vi "Cavities_State_v00.vi"(4 "BS Hold Pulse":bool, 6 "\"I too high?\"":T11, 11 "Control Cavity Cluster":T8={"Control A"={"Lock"=FALSE, "Hold"=FALSE, "P Gain"=0, "P BS"=-5, "I Gain"=0, "I BS"=-10, "I2 G"=0, "I2 BS"=-26, "Scan Amp"=0, "Scan Off"=0, "Scan FS"=0, "SFS BS"=0, "I Max value"=10000, "I2 Max value"=10000, "Scope.Offset"=0, "Trigger Direction"=enum."either", "Scan-PII thresh"=0}, "Control B"={"Lock"=FALSE, "Hold"=FALSE, "P Gain"=0, "P BS"=-5, "I Gain"=0, "I BS"=-10, "I2 G"=0, "I2 BS"=-26, "Scan Amp"=0, "Scan Off"=0, "Scan FS"=0, "SFS BS"=0, "I Max value"=10000, "I2 Max value"=10000, "Scope.Offset"=0, "Trigger Direction"=enum."either", "Scan-PII thresh"=0}, "Control MCC"={"Lock"=FALSE, "Hold"=FALSE, "P Gain"=0, "P BS"=-5, "I Gain"=0, "I BS"=-10, "I2 G"=0, "I2 BS"=-26, "Scan Amp"=0, "Scan Off"=0, "Scan FS"=0, "SFS BS"=0, "I Max value"=10000, "I2 Max value"=10000, "Scope.Offset"=0, "Trigger Direction"=enum."either", "Scan-PII thresh"=0}, "Control Doubler"={"Lock"=FALSE, "Hold"=FALSE, "P Gain"=0, "P BS"=-5, "I Gain"=0, "I BS"=-10, "I2 G"=0, "I2 BS"=-26, "Scan Amp"=0, "Scan Off"=0, "Scan FS"=0, "SFS BS"=0, "I Max value"=10000, "I2 Max value"=10000, "Scope.Offset"=0, "Trigger Direction"=enum."either", "Scan-PII thresh"=0}, "Lock Point?"={"OPO A"=FALSE, "OPO B"=FALSE, "MCC"=FALSE, "Doubler"=FALSE}, "Re-scan?"={"OPO A"=FALSE, "OPO B"=FALSE, "MCC"=FALSE, "Doubler"=FALSE}, "Cavity Errors"={"OPO A"=0, "OPO B"=0, "MCC"=0, "Doubler"=0}, "Max"={"Max OPO A"=0, "Max OPO B"=0, "Max MCC"=0, "Max Doubler"=0}, "Min"={"Min OPO A"=0, "Min OPO B"=0, "Min MCC"=0, "Min Doubler"=0}, "Lock Threshold"={"Thresh OPO A "=0, "Thresh OPO B"=0, "Thresh MCC"=0, "Thresh Doubler"=0}, "Re-Scan Threshold"={"Thresh OPO A "=0, "Thresh OPO B"=0, "Thresh MCC"=0, "Thresh Doubler"=0}, "State (-1)"={"OPO A"=enum."Safe", "OPO B"=enum."Safe", "MCC"=enum."Safe", "Doubler"=enum."Safe"}, "Lock pressed? (-1)"={"OPO A"=FALSE, "OPO B"=FALSE, "MCC"=FALSE, "Doubler"=FALSE}, "Safety First"={"lim reset"=FALSE, "no limit"=FALSE, "pos slew rate * dt"=0, "neg slew rate * dt"=0, "Hold All"=FALSE, "Count(Ticks)"=0}}) -> (3 "PII Scan State Errors":T5={"Control A"={"Lock"=FALSE, "Hold"=FALSE, "P Gain"=3, "P BS"=0, "I Gain"=0, "I BS"=-10, "I2 G"=0, "I2 BS"=-26, "Scan Amp"=0, "Scan Off"=0, "Scan FS"=0, "SFS BS"=0, "I Max value"=10000, "I2 Max value"=10000, "Scope.Offset"=0, "Trigger Direction"=enum."either", "Scan-PII thresh"=0}, "Control B"={"Lock"=FALSE, "Hold"=FALSE, "P Gain"=0, "P BS"=-5, "I Gain"=0, "I BS"=-10, "I2 G"=0, "I2 BS"=-26, "Scan Amp"=0, "Scan Off"=0, "Scan FS"=0, "SFS BS"=0, "I Max value"=10000, "I2 Max value"=10000, "Scope.Offset"=0, "Trigger Direction"=enum."either", "Scan-PII thresh"=0}, "Control MCC"={"Lock"=FALSE, "Hold"=FALSE, "P Gain"=0, "P BS"=-5, "I Gain"=0, "I BS"=-10, "I2 G"=0, "I2 BS"=-26, "Scan Amp"=0, "Scan Off"=0, "Scan FS"=0, "SFS BS"=0, "I Max value"=10000, "I2 Max value"=10000, "Scope.Offset"=0, "Trigger Direction"=enum."either", "Scan-PII thresh"=0}, "Control Doubler"={"Lock"=FALSE, "Hold"=FALSE, "P Gain"=0, "P BS"=-5, "I Gain"=0, "I BS"=-10, "I2 G"=0, "I2 BS"=-26, "Scan Amp"=0, "Scan Off"=0, "Scan FS"=0, "SFS BS"=0, "I Max value"=10000, "I2 Max value"=10000, "Scope.Offset"=0, "Trigger Direction"=enum."either", "Scan-PII thresh"=0}, "Cavity Errors"={"OPO A"=0, "OPO B"=0, "MCC"=0, "Doubler"=0}, "State"={"OPO A"=enum."Safe", "OPO B"=enum."Safe", "MCC"=enum."Safe", "Doubler"=enum."Safe"}}, 5 "MaxMin":T1)   [LabVIEW 2010]
doc: "The state of the output is decided here. There are four possible states: 1) Safe - zeros; 2) Hold - constant output of last value; 3) Scan - saw tooth at low frequency 4) Lock - PII output."
uses:
  Strict Type Defs/PII Scan State.ctl
  Strict Type Defs/PII individual.ctl
  Strict Type Defs/Cavity Errors.ctl
  Strict Type Defs/Control Cavity Cluster.ctl
  Strict Type Defs/Lock Point.ctl
  Strict Type Defs/Re-Scan.ctl
  Strict Type Defs/Max.ctl
  Strict Type Defs/Min.ctl
  Strict Type Defs/Safety First.ctl
  Strict Type Defs/MaxMin.ctl
panel:
  in  "MaxMin typedef":T1
  in  "Lock?":T11
  in  "PII Scan State":T5={"Control A"={"Lock"=FALSE, "Hold"=FALSE, "P Gain"=3, "P BS"=0, "I Gain"=0, "I BS"=-10, "I2 G"=0, "I2 BS"=-26, "Scan Amp"=0, "Scan Off"=0, "Scan FS"=0, "SFS BS"=0, "I Max value"=10000, "I2 Max value"=10000, "Scope.Offset"=0, "Trigger Direction"=enum."either", "Scan-PII thresh"=0}, "Control B"={"Lock"=FALSE, "Hold"=FALSE, "P Gain"=0, "P BS"=-5, "I Gain"=0, "I BS"=-10, "I2 G"=0, "I2 BS"=-26, "Scan Amp"=0, "Scan Off"=0, "Scan FS"=0, "SFS BS"=0, "I Max value"=10000, "I2 Max value"=10000, "Scope.Offset"=0, "Trigger Direction"=enum."either", "Scan-PII thresh"=0}, "Control MCC"={"Lock"=FALSE, "Hold"=FALSE, "P Gain"=0, "P BS"=-5, "I Gain"=0, "I BS"=-10, "I2 G"=0, "I2 BS"=-26, "Scan Amp"=0, "Scan Off"=0, "Scan FS"=0, "SFS BS"=0, "I Max value"=10000, "I2 Max value"=10000, "Scope.Offset"=0, "Trigger Direction"=enum."either", "Scan-PII thresh"=0}, "Control Doubler"={"Lock"=FALSE, "Hold"=FALSE, "P Gain"=0, "P BS"=-5, "I Gain"=0, "I BS"=-10, "I2 G"=0, "I2 BS"=-26, "Scan Amp"=0, "Scan Off"=0, "Scan FS"=0, "SFS BS"=0, "I Max value"=10000, "I2 Max value"=10000, "Scope.Offset"=0, "Trigger Direction"=enum."either", "Scan-PII thresh"=0}, "Cavity Errors"={"OPO A"=0, "OPO B"=0, "MCC"=0, "Doubler"=0}, "State"={"OPO A"=enum."Safe", "OPO B"=enum."Safe", "MCC"=enum."Safe", "Doubler"=enum."Safe"}}
  in  "State":T12
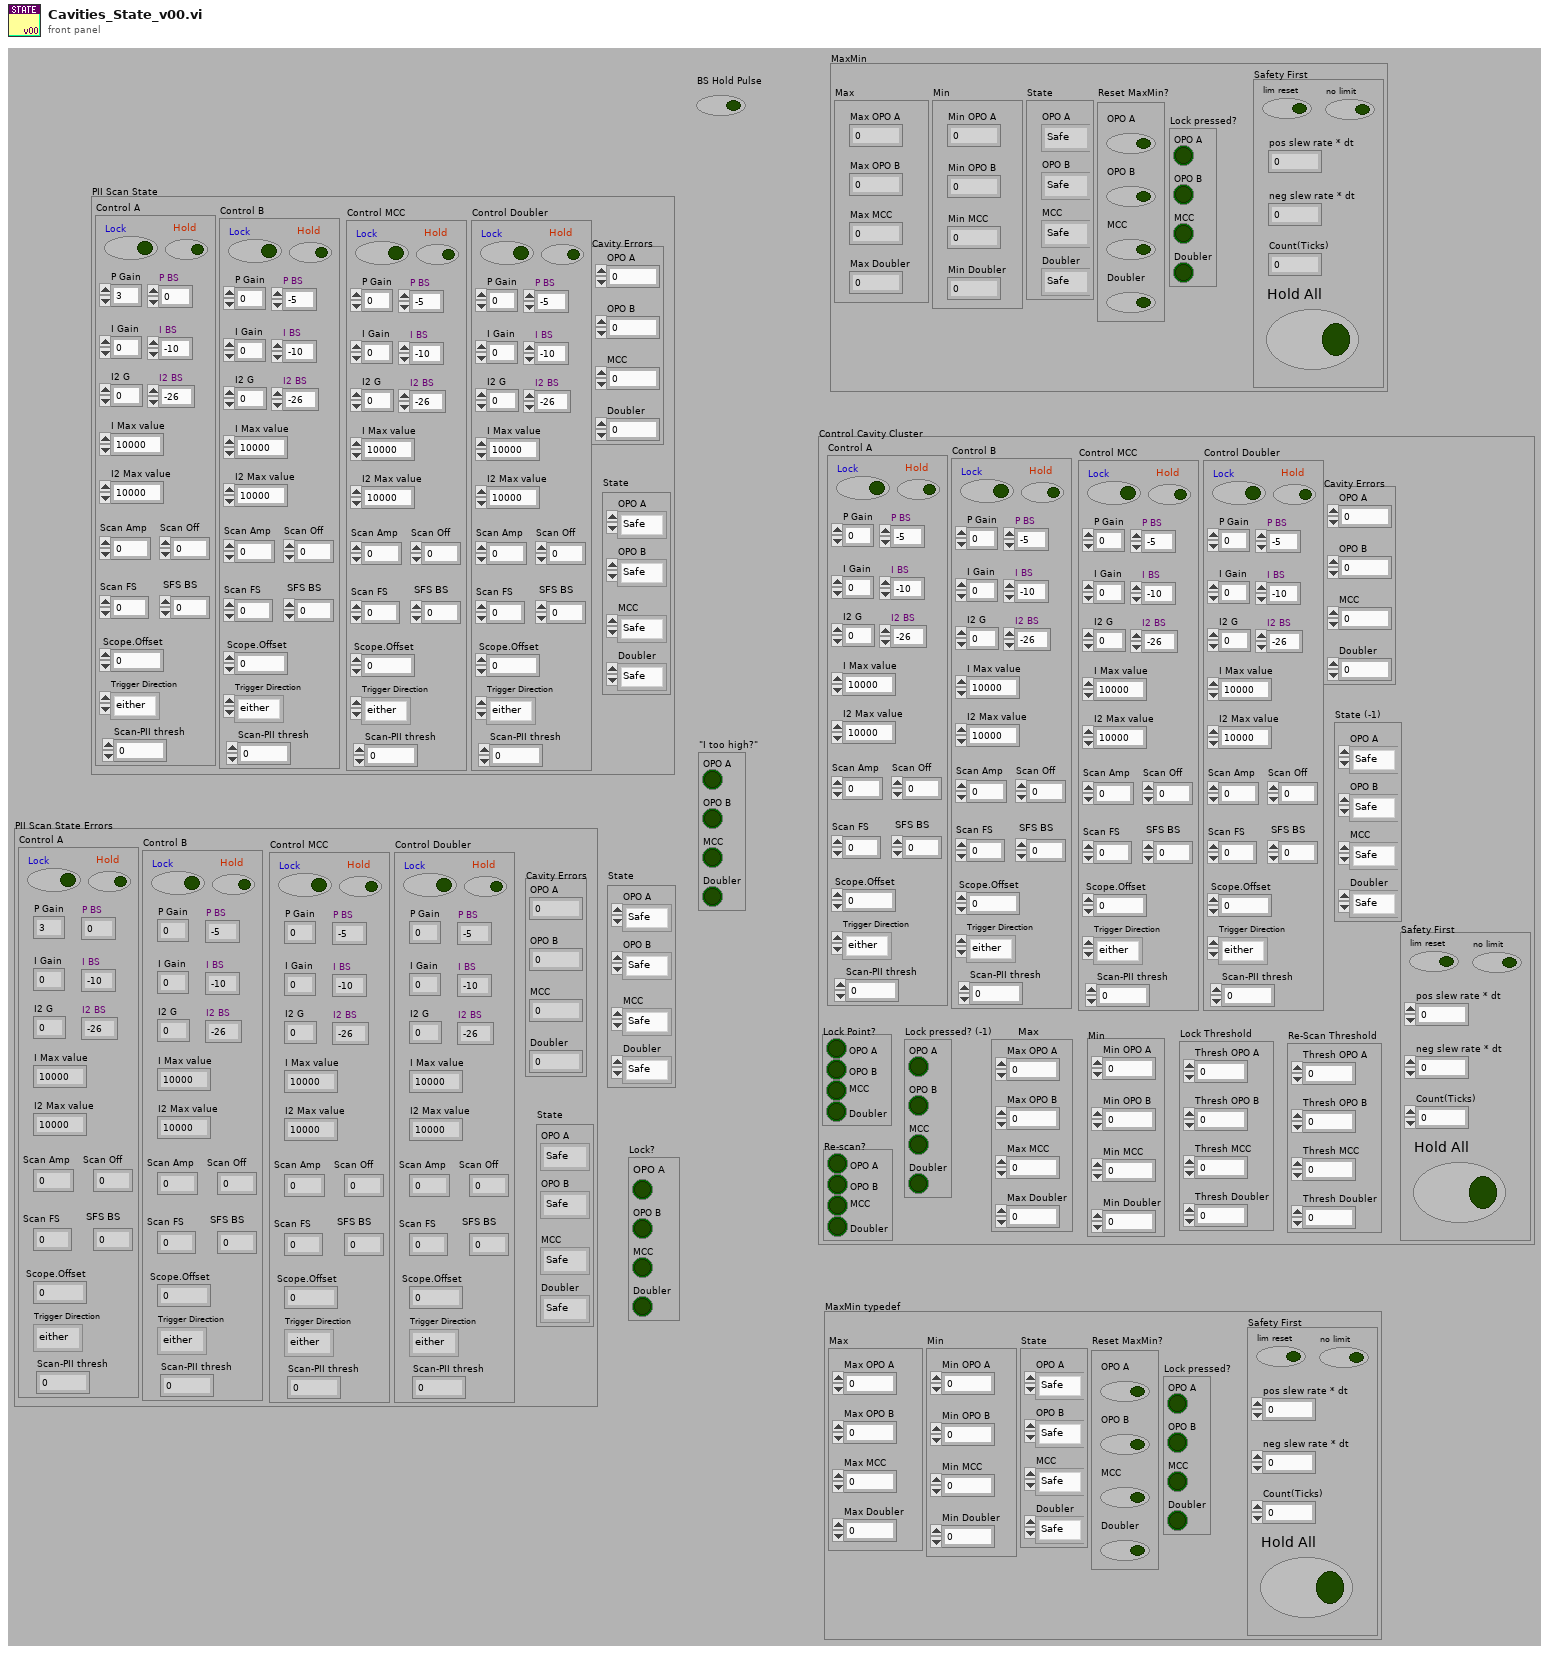
[diagram p1: front panel]
types:
  T1 = typedef "MaxMin.ctl" = cluster{"State":cluster{"OPO A":enum16{"Safe", "Hold", "Scan", "Lock"}, "OPO B":enum16{"Safe", "Hold", "Scan", "Lock"}, "MCC":enum16{"Safe", "Hold", "Scan", "Lock"}, "Doubler":enum16{"Safe", "Hold", "Scan", "Lock"}}, "Reset MaxMin?":cluster{"OPO A":bool, "OPO B":bool, "MCC":bool, "Doubler":bool}, "Max":T2, "Min":T3, "Lock pressed?":cluster{"OPO A":bool, "OPO B":bool, "MCC":bool, "Doubler":bool}, "Safety First":T4}
  T2 = typedef "Max.ctl" = cluster{"Max OPO A":i16, "Max OPO B":i16, "Max MCC":i16, "Max Doubler":i16}
  T3 = typedef "Min.ctl" = cluster{"Min OPO A":i16, "Min OPO B":i16, "Min MCC":i16, "Min Doubler":i16}
  T4 = typedef "Safety First.ctl" = cluster{"lim reset":bool, "no limit":bool, "pos slew rate * dt":i16, "neg slew rate * dt":i16, "Hold All":bool, "Count(Ticks)":u32}
  T5 = typedef "PII Scan State.ctl" = cluster{"Control A":T6, "Control B":T6, "Control MCC":T6, "Control Doubler":T6, "Cavity Errors":T7, "State":cluster{"OPO A":enum16{"Safe", "Hold", "Scan", "Lock"}, "OPO B":enum16{"Safe", "Hold", "Scan", "Lock"}, "MCC":enum16{"Safe", "Hold", "Scan", "Lock"}, "Doubler":enum16{"Safe", "Hold", "Scan", "Lock"}}}
  T6 = typedef "PII individual.ctl" = cluster{"Lock":bool, "Hold":bool, "P Gain":i32, "P BS":i16, "I Gain":i32, "I BS":i16, "I2 G":i32, "I2 BS":i16, "Scan Amp":i16, "Scan Off":i16, "Scan FS":u16, "SFS BS":i16, "I Max value":i32, "I2 Max value":i32, "Scope.Offset":i16, "Trigger Direction":enum8{"either", "minus-plus", "plus-minus"}, "Scan-PII thresh":i16}
  T7 = typedef "Cavity Errors.ctl" = cluster{"OPO A":i16, "OPO B":i16, "MCC":i16, "Doubler":i16}
  T8 = typedef "Control Cavity Cluster.ctl" = cluster{"Control A":T6, "Control B":T6, "Control MCC":T6, "Control Doubler":T6, "Lock Point?":T9, "Re-scan?":T10, "Cavity Errors":T7, "Max":T2, "Min":T3, "Lock Threshold":cluster{"Thresh OPO A ":i16, "Thresh OPO B":i16, "Thresh MCC":i16, "Thresh Doubler":i16}, "Re-Scan Threshold":cluster{"Thresh OPO A ":i16, "Thresh OPO B":i16, "Thresh MCC":i16, "Thresh Doubler":i16}, "State (-1)":cluster{"OPO A":enum16{"Safe", "Hold", "Scan", "Lock"}, "OPO B":enum16{"Safe", "Hold", "Scan", "Lock"}, "MCC":enum16{"Safe", "Hold", "Scan", "Lock"}, "Doubler":enum16{"Safe", "Hold", "Scan", "Lock"}}, "Lock pressed? (-1)":cluster{"OPO A":bool, "OPO B":bool, "MCC":bool, "Doubler":bool}, "Safety First":T4}
  T9 = typedef "Lock Point.ctl" = cluster{"OPO A":bool, "OPO B":bool, "MCC":bool, "Doubler":bool}
  T10 = typedef "Re-Scan.ctl" = cluster{"OPO A":bool, "OPO B":bool, "MCC":bool, "Doubler":bool}
  T11 = cluster{"OPO A":bool, "OPO B":bool, "MCC":bool, "Doubler":bool}
  T12 = cluster{"OPO A":enum16{"Safe", "Hold", "Scan", "Lock"}, "OPO B":enum16{"Safe", "Hold", "Scan", "Lock"}, "MCC":enum16{"Safe", "Hold", "Scan", "Lock"}, "Doubler":enum16{"Safe", "Hold", "Scan", "Lock"}}
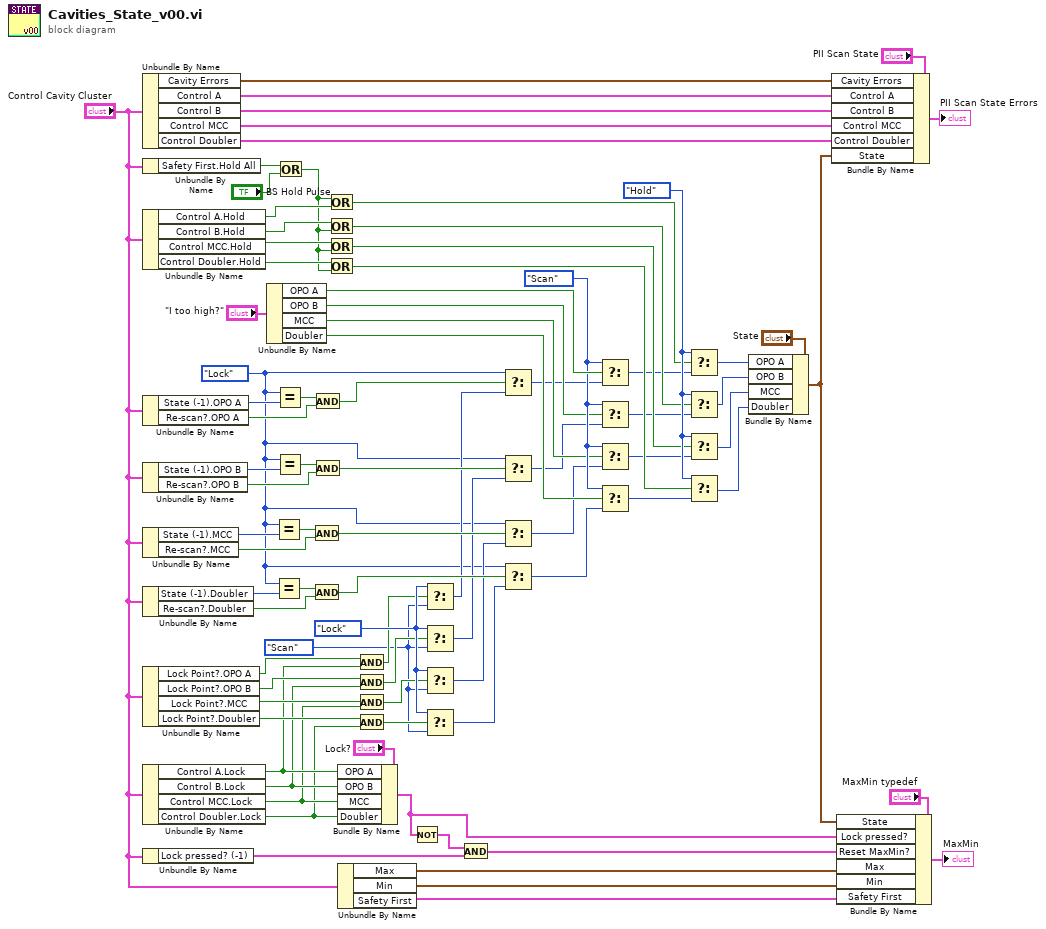
[diagram p0: block diagram]
diagram:
  w56 = enum16{"Safe", "Hold", "Scan", "Lock"}."Scan" ("State")
  w1 = enum16{"Safe", "Hold", "Scan", "Lock"}."Lock" ("y")
  w76 = enum16{"Safe", "Hold", "Scan", "Lock"}."Hold" ("State")
  w70 = enum16{"Safe", "Hold", "Scan", "Lock"}."Scan" ("State")
  w85 = enum16{"Safe", "Hold", "Scan", "Lock"}."Lock" ("State")
  n1 = Unbundle By Name("Control Cavity Cluster") -> ("Cavity Errors"=w55:T7, "Control A"=w54:T6, "Control B"=w53:T6, "Control MCC"=w52:T6, "Control Doubler"=w51:T6)
  n2 = Unbundle By Name("Control Cavity Cluster") -> ("Safety First.Hold All"=w5:bool)
  n3 = Unbundle By Name("Control Cavity Cluster") -> ("Control A.Hold"=w75:bool, "Control B.Hold"=w39:bool, "Control MCC.Hold"=w38:bool, "Control Doubler.Hold"=w37:bool)
  n4 = Unbundle By Name("Control Cavity Cluster") -> ("State (-1).OPO A"=w25:enum16{"Safe", "Hold", "Scan", "Lock"}, "Re-scan?.OPO A"=w67:bool)
  n5 = Unbundle By Name("Control Cavity Cluster") -> ("State (-1).OPO B"=w26:enum16{"Safe", "Hold", "Scan", "Lock"}, "Re-scan?.OPO B"=w66:bool)
  n6 = Unbundle By Name("Control Cavity Cluster") -> ("State (-1).MCC"=w27:enum16{"Safe", "Hold", "Scan", "Lock"}, "Re-scan?.MCC"=w60:bool)
  n7 = Unbundle By Name("Control Cavity Cluster") -> ("State (-1).Doubler"=w28:enum16{"Safe", "Hold", "Scan", "Lock"}, "Re-scan?.Doubler"=w61:bool)
  n8 = Unbundle By Name("Control Cavity Cluster") -> ("Lock Point?.OPO A"=w36:bool, "Lock Point?.OPO B"=w35:bool, "Lock Point?.MCC"=w34:bool, "Lock Point?.Doubler"=w33:bool)
  n9 = Unbundle By Name("Control Cavity Cluster") -> ("Control A.Lock"=w32:bool, "Control B.Lock"=w31:bool, "Control MCC.Lock"=w30:bool, "Control Doubler.Lock"=w29:bool)
  n10 = Unbundle By Name("Control Cavity Cluster") -> ("Lock pressed? (-1)"=w48:T11)
  n11 = Unbundle By Name("\"I too high?\"") -> ("OPO A"=w69:bool, "OPO B"=w43:bool, "MCC"=w42:bool, "Doubler"=w41:bool)
  n12 = Equal?(x=w1, y=w27) -> (x = y?=w59:bool)
  n13 = Equal?(x=w1, y=w28) -> (x = y?=w62:bool)
  n14 = Equal?(x=w1, y=w25) -> (x = y?=w68:bool)
  n15 = Equal?(x=w1, y=w26) -> (x = y?=w65:bool)
  n16 = Or(x=w5, y="BS Hold Pulse") -> (x .or. y?=w3:bool)
  n17 = And(x=w59, y=w60) -> (x .and. y?=w58:bool)
  n18 = And(x=w62, y=w61) -> (x .and. y?=w63:bool)
  n19 = And(x=w68, y=w67) -> (x .and. y?=w77:bool)
  n20 = And(x=w65, y=w66) -> (x .and. y?=w64:bool)
  n21 = Or(x=w3, y=w75) -> (x .or. y?=w74:bool)
  n22 = Or(x=w39, y=w3) -> (x .or. y?=w73:bool)
  n23 = Or(x=w38, y=w3) -> (x .or. y?=w72:bool)
  n24 = Or(x=w37, y=w3) -> (x .or. y?=w71:bool)
  n25 = Bundle By Name(cluster="Lock?", "OPO A"=w32, "OPO B"=w31, "MCC"=w30, "Doubler"=w29) -> (w2:T11)
  n26 = Unbundle By Name("Control Cavity Cluster") -> ("Max"=w24:T2, "Min"=w23:T3, "Safety First"=w22:T4)
  n27 = And(x=w36, y=w32) -> (x .and. y?=w79:bool)
  n28 = And(x=w35, y=w31) -> (x .and. y?=w80:bool)
  n29 = And(x=w34, y=w30) -> (x .and. y?=w81:bool)
  n30 = And(x=w33, y=w29) -> (x .and. y?=w82:bool)
  n31 = Not(x=w2) -> (.not. x?=w57:T11)
  n32 = Select(t=w85, s=w79, f=w70) -> (s? t:f=w21:enum16{"Safe", "Hold", "Scan", "Lock"})
  n33 = Select(t=w85, s=w80, f=w70) -> (s? t:f=w20:enum16{"Safe", "Hold", "Scan", "Lock"})
  n34 = Select(t=w85, s=w81, f=w70) -> (s? t:f=w19:enum16{"Safe", "Hold", "Scan", "Lock"})
  n35 = Select(t=w85, s=w82, f=w70) -> (s? t:f=w18:enum16{"Safe", "Hold", "Scan", "Lock"})
  n36 = And(x=w57, y=w48) -> (x .and. y?=w46:T11)
  n37 = Select(t=w1, s=w77, f=w21) -> (s? t:f=w17:enum16{"Safe", "Hold", "Scan", "Lock"})
  n38 = Select(t=w1, s=w64, f=w20) -> (s? t:f=w16:enum16{"Safe", "Hold", "Scan", "Lock"})
  n39 = Select(t=w1, s=w58, f=w19) -> (s? t:f=w15:enum16{"Safe", "Hold", "Scan", "Lock"})
  n40 = Select(t=w1, s=w63, f=w18) -> (s? t:f=w14:enum16{"Safe", "Hold", "Scan", "Lock"})
  n41 = Select(t=w56, s=w69, f=w17) -> (s? t:f=w13:enum16{"Safe", "Hold", "Scan", "Lock"})
  n42 = Select(t=w56, s=w43, f=w16) -> (s? t:f=w12:enum16{"Safe", "Hold", "Scan", "Lock"})
  n43 = Select(t=w56, s=w42, f=w15) -> (s? t:f=w11:enum16{"Safe", "Hold", "Scan", "Lock"})
  n44 = Select(t=w56, s=w41, f=w14) -> (s? t:f=w10:enum16{"Safe", "Hold", "Scan", "Lock"})
  n45 = Select(t=w76, s=w74, f=w13) -> (s? t:f=w9:enum16{"Safe", "Hold", "Scan", "Lock"})
  n46 = Select(t=w76, s=w73, f=w12) -> (s? t:f=w8:enum16{"Safe", "Hold", "Scan", "Lock"})
  n47 = Select(t=w76, s=w72, f=w11) -> (s? t:f=w7:enum16{"Safe", "Hold", "Scan", "Lock"})
  n48 = Select(t=w76, s=w71, f=w10) -> (s? t:f=w6:enum16{"Safe", "Hold", "Scan", "Lock"})
  n49 = Bundle By Name(cluster="State", "OPO A"=w9, "OPO B"=w8, "MCC"=w7, "Doubler"=w6) -> (w45:T12)
  n50 = Bundle By Name(cluster="PII Scan State", "Cavity Errors"=w55, "Control A"=w54, "Control B"=w53, "Control MCC"=w52, "Control Doubler"=w51, "State"=w45) -> (→"PII Scan State Errors":T5)
  n51 = Bundle By Name(cluster="MaxMin typedef", "State"=w45, "Lock pressed?"=w2, "Reset MaxMin?"=w46, "Max"=w24, "Min"=w23, "Safety First"=w22) -> (→"MaxMin":T1)
